vi "example_data_raw_pipeline.vi"() -> ()   [LabVIEW 2020]
uses:
  src/data/data_node/data_node.lvclass
  D:/Personal/LabVIEW LLMs/src/data/abstract_data_base/abstract_data_base.lvclass
  src/data/data_document/data_document.lvclass
  src/vectorstore/vector_qdrant/vector_qdrant.lvclass
  D:/Personal/LabVIEW LLMs/src/vectorstore/abstract_vector_base/abstract_vector_base.lvclass
  src/models/llm_openai_embedding/llm_openai_embedding.lvclass
  D:/Personal/LabVIEW LLMs/src/models/abstract_llm_base/abstract_llm_base.lvclass
  src/models/llm_openai_embedding/Instantiate_llm_openai_embed.vi
  src/data_processor/chunk_character_splitter/chunk_character_splitter.lvclass
  src/data_source/datasource_text_file/datasource_text_file.lvclass
  src/data_destination/destination_vectorstore/destination_vectorstore.lvclass
  src/data_processor/embed_nodes/embed_nodes.lvclass
  src/utilities/env_variables/env_variables.lvlib
panel:
  in  "max_character_length":u32=500
  in  "recursive_folder_load":bool
  in  "model_name":string(combo)="text-embedding-ada-002"
  out "embed nodes":refnum<class "data_node.lvclass">[](array[class])
  out "source document":refnum<class "data_document.lvclass">[](array[class])
  out "chunk nodes":refnum<class "data_node.lvclass">[](array[class])
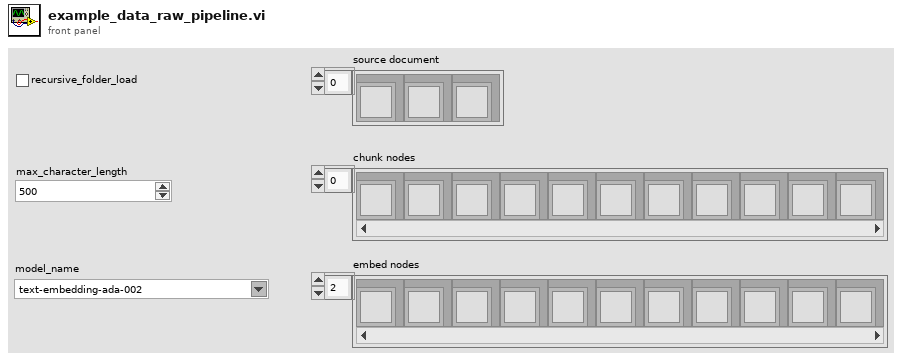
[diagram p1: front panel]
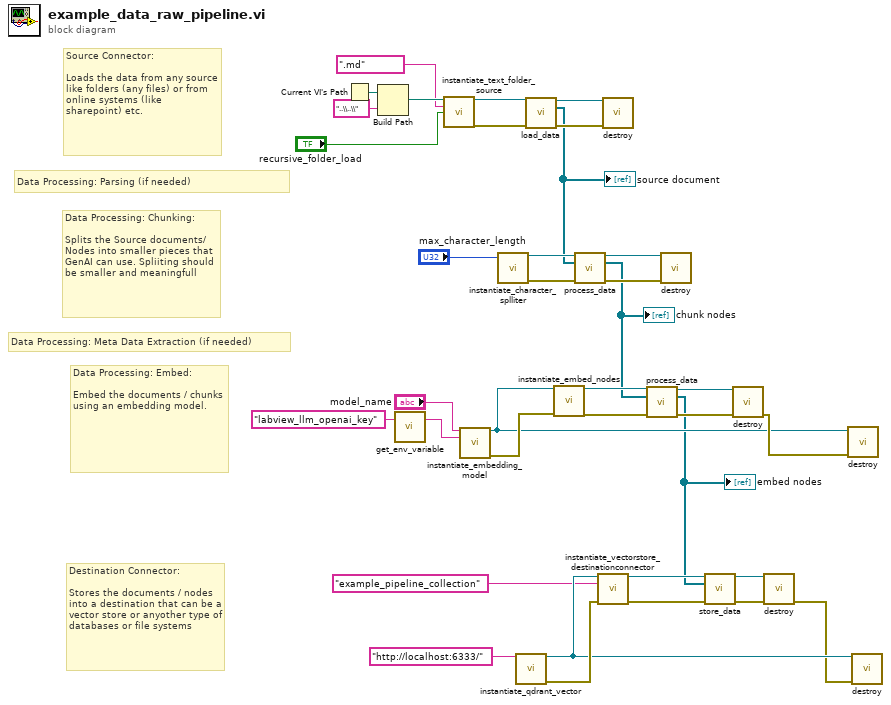
[diagram p0: block diagram]
diagram:
  # "Destination Connector:\n\nStores the documents / nodes into a destination that can be a vector store or anyother type of databases or file systems"
  # "Data Processing: Meta Data Extraction (if needed)"
  # "Data Processing: Parsing (if needed)"
  # "Data Processing: Embed:\n\nEmbed the documents / chunks using an embedding model."
  # "Data Processing: Chunking:\n\nSplits the Source documents/Nodes into smaller pieces that GenAI can use. Spliiting should be smaller and meaningfull"
  # "Source Connector:\n\nLoads the data from any source like folders (any files) or from online systems (like sharepoint) etc."
  n1 = Current VI's Path() -> (path=w36:path)
  n2 = Build Path(base path=w36, name or relative path="..\\..\\") -> (appended path=w34:path)
  n3 = call "get_env_variable.vi"("Environment Variable Name"="labview_llm_openai_key") -> ("Value"=w15:string)  [unwired: 1 in, 1 out]
  n4 = call "instantiate_text_folder_source.vi"("source_folder"=w34, "file_extension"=".md", "recursive_folder_load"="recursive_folder_load") -> ("datasource_text_file out"=w32:refnum<class "datasource_text_file.lvclass">, "error out"=w31:errorcluster)  [unwired: 11 in]
  n5 = call-poly "instantiate_embedding_model.vi"("model_name"="model_name", "openai_key"=w15) -> ("llm_openai_embedding out"=w12:refnum<class "llm_openai_embedding.lvclass">, "error out"=w14:errorcluster)  [unwired: 12 in]
  n6 = call "instantiate_character_splliter.vi"("max_character_length"="max_character_length") -> ("chunk_character_splitter out"=w27:refnum<class "chunk_character_splitter.lvclass">, "error out"=w26:errorcluster)  [unwired: 13 in]
  n7 = call "instantiate_qdrant_vector.vi"("host_url"="http://localhost:6333/") -> ("vector_qdrant out"=w9:refnum<class "vector_qdrant.lvclass">, "error out"=w10:errorcluster)  [unwired: 13 in]
  n8 = call-dynamic "load_data.vi"("datasource_text_file in"=w32, "error in (no error)"=w31) -> ("datasource_text_file out"=w30:refnum<class "datasource_text_file.lvclass">, "document"=w23:refnum<class "data_document.lvclass">[], "error out"=w29:errorcluster)  [unwired: 11 in]
  "source document" <- w23
  n9 = call "instantiate_embed_nodes.vi"("abstract_llm_embedding"=w12, "error in (no error)"=w14) -> ("embed_nodes out"=w22:refnum<class "embed_nodes.lvclass">, "error out"=w21:errorcluster)  [unwired: 12 in]
  n10 = call-dynamic "process_data.vi"("abstract_dataprocessing_base in"=w27, "datas"=w23, "error in (no error)"=w26) -> ("abstract_dataprocessing_base out"=w25:refnum<class "chunk_character_splitter.lvclass">, "nodes"=w18:refnum<class "data_node.lvclass">[], "error out"=w24:errorcluster)  [unwired: 10 in]
  "chunk nodes" <- w18
  n11 = call "instantiate_vectorstore_destinationconnector.vi"("abstract_vector_base"=w9, "store_id"="example_pipeline_collection", "error in (no error)"=w10) -> ("destination_vectorstore out"=w8:refnum<class "destination_vectorstore.lvclass">, "error out"=w7:errorcluster)  [unwired: 11 in]
  n12 = call-dynamic "destroy.vi"("abstract_datasource_base in"=w30, "error in (no error)"=w29) -> ()  [unwired: 12 in, 2 out]
  n13 = call-dynamic "process_data.vi"("abstract_dataprocessing_base in"=w22, "datas"=w18, "error in (no error)"=w21) -> ("abstract_dataprocessing_base out"=w19:refnum<class "embed_nodes.lvclass">, "nodes"=w6:refnum<class "data_node.lvclass">[], "error out"=w20:errorcluster)  [unwired: 10 in]
  "embed nodes" <- w6
  n14 = call-dynamic "destroy.vi"("abstract_dataprocessing_base in"=w25, "error in (no error)"=w24) -> ()  [unwired: 12 in, 2 out]
  n15 = call-dynamic "store_data.vi"("abstract_datadestination_base in"=w8, "datas"=w6, "error in (no error)"=w7) -> ("abstract_datadestination_base out"=w5:refnum<class "destination_vectorstore.lvclass">, "error out"=w4:errorcluster)  [unwired: 11 in]
  n16 = call-dynamic "destroy.vi"("abstract_dataprocessing_base in"=w19, "error in (no error)"=w20) -> ("error out"=w13:errorcluster)  [unwired: 12 in, 1 out]
  n17 = call-dynamic "destroy.vi"("abstract_datadestination_base in"=w5, "error in (no error)"=w4) -> ("error out"=w3:errorcluster)  [unwired: 12 in, 1 out]
  n18 = call-dynamic "destroy.vi"("error in (no error)"=w13, "llm_openai_embedding in"=w12) -> ()  [unwired: 8 in, 2 out]
  n19 = call-dynamic "destroy.vi"("vector_qdrant in"=w9, "error in (no error)"=w3) -> ()  [unwired: 12 in, 2 out]
